vi "Write Connection Number.vi"(8 "error in (no error)":errorcluster, 10 "Connection Number":i32, 11 "TCP_Client_Window in":refnum<class "TCP_Client_Window.lvclass">) -> (0 "error out":errorcluster, 3 "TCP_Client_Window out":refnum<class "TCP_Client_Window.lvclass">)   [LabVIEW 2023, in "TCP_Client_Window.lvlib" / "TCP_Client_Window.lvclass"]
uses:
  TCP_Client_Window.lvclass
  TCP_Client_Window.lvclass/TCP_Client_Window.ctl
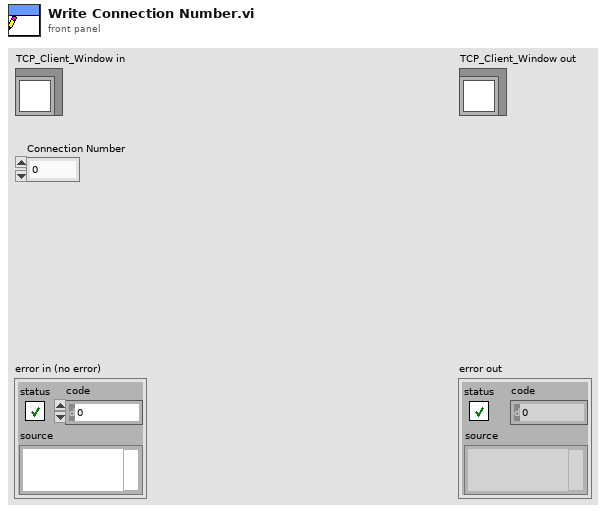
[diagram p1: front panel]
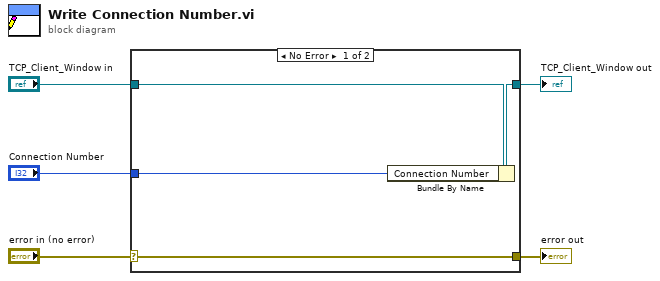
[diagram p0: block diagram]
diagram:
  n1 = case shown="No Error" "error in (no error)" {
    selector: "error in (no error)" -> [w9 w10]
    tunnel: [w9 w10] -> w4
    tunnel: [w7 w11] -> w2
    tunnel: "TCP_Client_Window in" -> [w8 w11]
    tunnel: "Connection Number" -> [w6 _]
    frame No Error {
      n2 = Bundle By Name(cluster=w8, "Connection Number"=w6) -> (w7:refnum<class "TCP_Client_Window.lvclass">)
    }
    frame Error {
    }
  }
  "error out" <- w4
  "TCP_Client_Window out" <- w2
